vi "Tutorial 6.vi"() -> ()   [LabVIEW 2022 SP3]
panel:
  in  "User input list":string
  out "Array - String":string[](array[string])
  in  "function name":string
  in  "Python version":string
  in  "stop":bool
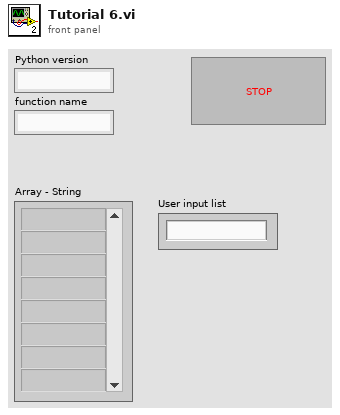
[diagram p1: front panel]
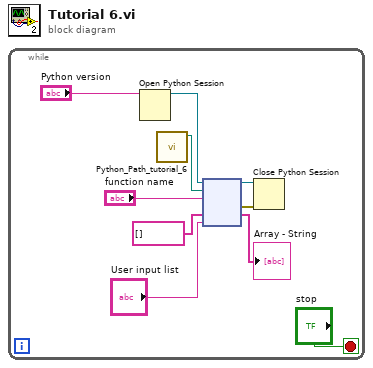
[diagram p0: block diagram]
diagram:
  n1 = while {
    stop <- "stop" stop-if-true
    n2 = Open Python Session(python version="Python version") -> (session out=w8:refnum<k35>)  [unwired: 2 in, 1 out]
    n3 = call "Python_Path_tutorial_6.vi"() -> ("appended path"=w5:path)  [unwired: 11 in]
    n4 = node(w8, w5, "function name", string[] [], "User input list") -> (w7:refnum<k35>, w6:errorcluster, →"Array - String":string[])  [unwired: 2 in, 2 out]
    n5 = Close Python Session(session in=w7, error in=w6) -> ()  [unwired: 1 out]
  }
